vi "Authenticate.vi"(8 "error in (no error)":errorcluster, 9 "Refresh Token":string, 10 "Authentication Info":T1, 11 "Scope Needed?":T2) -> (0 "error out":errorcluster, 1 "Refresh Token":string, 2 "Timeout":dbl, 3 "Access Token":string)   [LabVIEW 2016]
uses:
  scope_needed.ctl
  OAuth/OAuth.lvclass
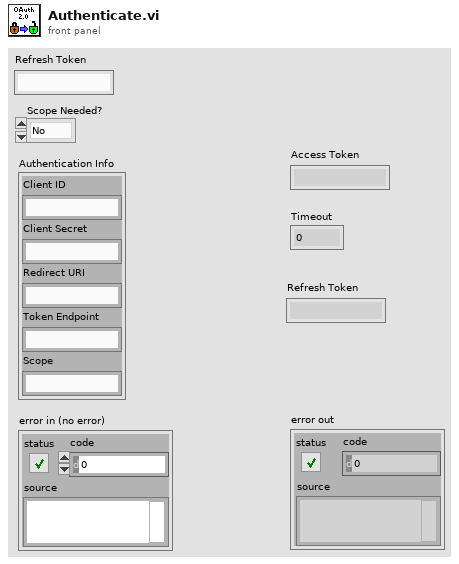
[diagram p1: front panel]
types:
  T1 = cluster{"Client ID":string, "Client Secret":string, "Redirect URI":string, "Token Endpoint":string, "Scope":string}
  T2 = typedef "scope_needed.ctl" = enum16{"No", "Yes"}
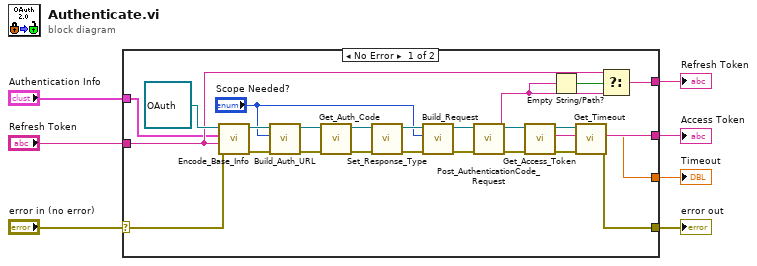
[diagram p0: block diagram]
diagram:
  n1 = case shown="No Error" "error in (no error)" {
    selector: "error in (no error)" -> [w32 w33]
    tunnel: [w24 w33] -> w6
    tunnel: [w23 _] -> w5
    tunnel: [w22 _] -> w4
    tunnel: [w10 _] -> w3
    tunnel: "Refresh Token" -> [w12 _]
    tunnel: "Authentication Info" -> [w8 _]
    frame No Error {
      n2 = call "Encode_Base_Info.vi"("error in (no error)"=w32, "Refresh Token"=w12, "Authentication Info"=w8, "OAuth in"=refnum<class "OAuth.lvclass"> refnum ("OAuth.lvclass")) -> ("error out"=w17:errorcluster, "OAuth out"=w15:refnum<class "OAuth.lvclass">)  [unwired: 6 in]
      n3 = call "Build_Auth_URL.vi"("error in (no error)"=w17, "Application"="Scope Needed?", "OAuth in"=w15) -> ("error out"=w16:errorcluster, "OAuth out"=w14:refnum<class "OAuth.lvclass">)  [unwired: 7 in]
      n4 = call-dynamic "Get_Auth_Code.vi"("error in (no error)"=w16, "OAuth in"=w14) -> ("error out"=w20:errorcluster, "OAuth out"=w21:refnum<class "OAuth.lvclass">)  [unwired: 8 in]
      n5 = call "Set_Response_Type.vi"("error in (no error)"=w20, "OAuth in"=w21) -> ("error out"=w19:errorcluster, "OAuth out"=w18:refnum<class "OAuth.lvclass">)  [unwired: 8 in]
      n6 = call-dynamic "Build_Request.vi"("error in (no error)"=w19, "Application"="Scope Needed?", "OAuth in"=w18) -> ("error out"=w29:errorcluster, "OAuth out"=w30:refnum<class "OAuth.lvclass">)  [unwired: 7 in]
      n7 = call-dynamic "Post_AuthenticationCode_Request.vi"("error in (no error)"=w29, "OAuth in"=w30) -> ("error out"=w28:errorcluster, "Refresh Token"=w9:string, "OAuth out"=w26:refnum<class "OAuth.lvclass">)  [unwired: 7 in]
      n8 = call-dynamic "Get_Access_Token.vi"("error in (no error)"=w28, "OAuth in"=w26) -> ("error out"=w27:errorcluster, "Access Token"=w23:string, "OAuth out"=w25:refnum<class "OAuth.lvclass">)  [unwired: 7 in]
      n9 = Empty String/Path?(string/path=w9) -> (empty?=w11:bool)
      n10 = call-dynamic "Get_Timeout.vi"("error in (no error)"=w27, "OAuth in"=w25) -> ("error out"=w24:errorcluster, "Timeout"=w22:dbl)  [unwired: 7 in, 1 out]
      n11 = Select(t=w12, s=w11, f=w9) -> (s? t:f=w10:string)
    }
    frame Error {
    }
  }
  "error out" <- w6
  "Access Token" <- w5
  "Timeout" <- w4
  "Refresh Token" <- w3
